vi "Close.vi"(8 "error in (no error)":errorcluster, 11 "LogicIO in":refnum<class "LogicIO.lvclass">) -> (0 "error out":errorcluster, 3 "LogicIO out":refnum<class "LogicIO.lvclass">)   [LabVIEW 2016, in "Hardware.lvlib" / "LogicIO.lvlib" / "LogicIO.lvclass"]
uses:
  <userlib>/Common Components/Hardware/LogicIO/LogicIO/LogicIO.lvclass
  <userlib>/Common Components/Hardware/LogicIO/LogicIO/LogicIO.lvclass/LogicIO.ctl
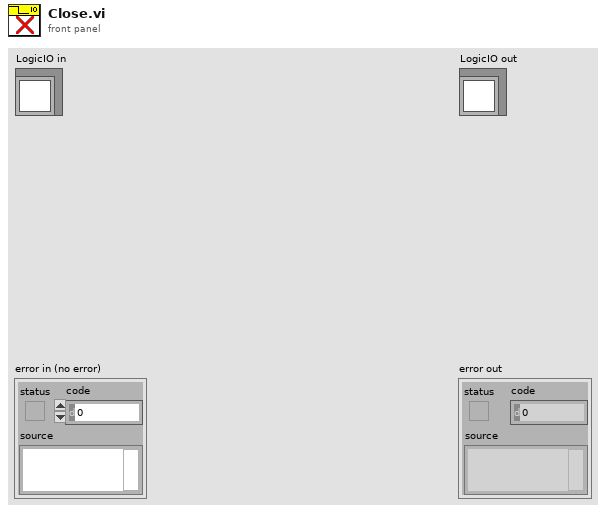
[diagram p1: front panel]
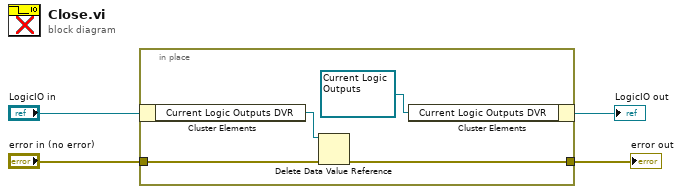
[diagram p0: block diagram]
diagram:
  n1 = in-place {
    in-place-border: "error in (no error)" -> [w8]
    in-place-border: [w7] -> w3
    n2 = in-place-cluster #1("LogicIO in") -> ("Current Logic Outputs DVR"=w6:refnum<data-value>)
    n3 = Delete Data Value Reference(data value reference=w6, error in=w8) -> (error out=w7:errorcluster)  [unwired: 1 out]
    n4 = in-place-cluster #1("Current Logic Outputs DVR"=refnum<data-value> refnum) -> (→"LogicIO out":refnum<class "LogicIO.lvclass">)
  }
  "error out" <- w3
